vi "ex_InitTabControl.vi"(3 "DAQmx properties tree for storage":refnum<vi>, 4 "Source":refnum<vi>, 7 "error in (no error)":errorcluster, 9 "Classes":T1[](array[typedef]) {"Events"."Event Code" max=1073741823 step=1 format="%x"; "Methods"."Method Code" format="%x"; "Attributes"."Number of Dimensions" format="%x"; "Attributes"."Property Code" format="%x"}) -> ()   [LabVIEW 2020, in "Configure User Def Prop.xctl"]
uses:
  <vilib>/Platform/express/ex_EditUserDefinedProperties/Configure User Def Prop.xctl
  <vilib>/Platform/express/ex_EditUserDefinedProperties/controls.llb/ex_class3.ctl
  <vilib>/Platform/express/ex_EditUserDefinedProperties/controls.llb/ex_generictype3.ctl
  <vilib>/Platform/express/ex_EditUserDefinedProperties/controls.llb/ex_refnumenum.ctl
  <vilib>/Platform/express/ex_EditUserDefinedProperties/controls.llb/ex_cleanupenum.ctl
  <vilib>/Platform/express/ex_EditUserDefinedProperties/controls.llb/ex_yesnodefaultenum.ctl
  <vilib>/Platform/express/ex_EditUserDefinedProperties/controls.llb/ex_errorpassingenum.ctl
  <vilib>/Platform/express/ex_EditUserDefinedProperties/controls.llb/ex_matchexactenum.ctl
  <vilib>/Platform/express/ex_EditUserDefinedProperties/controls.llb/ex_callingenum.ctl
  <vilib>/Platform/express/ex_EditUserDefinedProperties/controls.llb/ex_filtering.ctl
  <vilib>/Platform/express/ex_EditUserDefinedProperties/controls.llb/ex_dialogenum.ctl
  <vilib>/Platform/express/ex_EditUserDefinedProperties/controls.llb/ex_attribute3.ctl
  <vilib>/Platform/express/ex_EditUserDefinedProperties/controls.llb/ex_datatypeenum.ctl
  <vilib>/Platform/express/ex_EditUserDefinedProperties/controls.llb/ex_clustercontrol.ctl
  <vilib>/Platform/express/ex_EditUserDefinedProperties/controls.llb/ex_enumeration.ctl
  <vilib>/Platform/express/ex_EditUserDefinedProperties/controls.llb/ex_yesnoenum.ctl
  <vilib>/Platform/express/ex_EditUserDefinedProperties/controls.llb/ex_accessenum.ctl
  <vilib>/Platform/express/ex_EditUserDefinedProperties/controls.llb/ex_initnameformat.ctl
  <vilib>/Platform/express/ex_EditUserDefinedProperties/controls.llb/ex_method3.ctl
  <vilib>/Platform/express/ex_EditUserDefinedProperties/controls.llb/ex_methflagsenum.ctl
  <vilib>/Platform/express/ex_EditUserDefinedProperties/controls.llb/ex_parameter2.ctl
  <vilib>/Platform/express/ex_EditUserDefinedProperties/controls.llb/ex_datanameenum.ctl
  <vilib>/Platform/express/ex_EditUserDefinedProperties/controls.llb/ex_numericdatatypeenum.ctl
  <vilib>/Platform/express/ex_EditUserDefinedProperties/controls.llb/ex_stringdatatypeenum.ctl
  <vilib>/Platform/express/ex_EditUserDefinedProperties/controls.llb/ex_passbyenum.ctl
  <vilib>/Platform/express/ex_EditUserDefinedProperties/controls.llb/ex_arrayfmtenum.ctl
  <vilib>/Platform/express/ex_EditUserDefinedProperties/controls.llb/ex_paraminoutenum.ctl
  <vilib>/Platform/express/ex_EditUserDefinedProperties/controls.llb/ex_eventdef.ctl
  <vilib>/Platform/express/ex_EditUserDefinedProperties/controls.llb/ex_eventparam.ctl
  <vilib>/Platform/express/ex_EditUserDefinedProperties/controls.llb/ex_eventparamtype.ctl
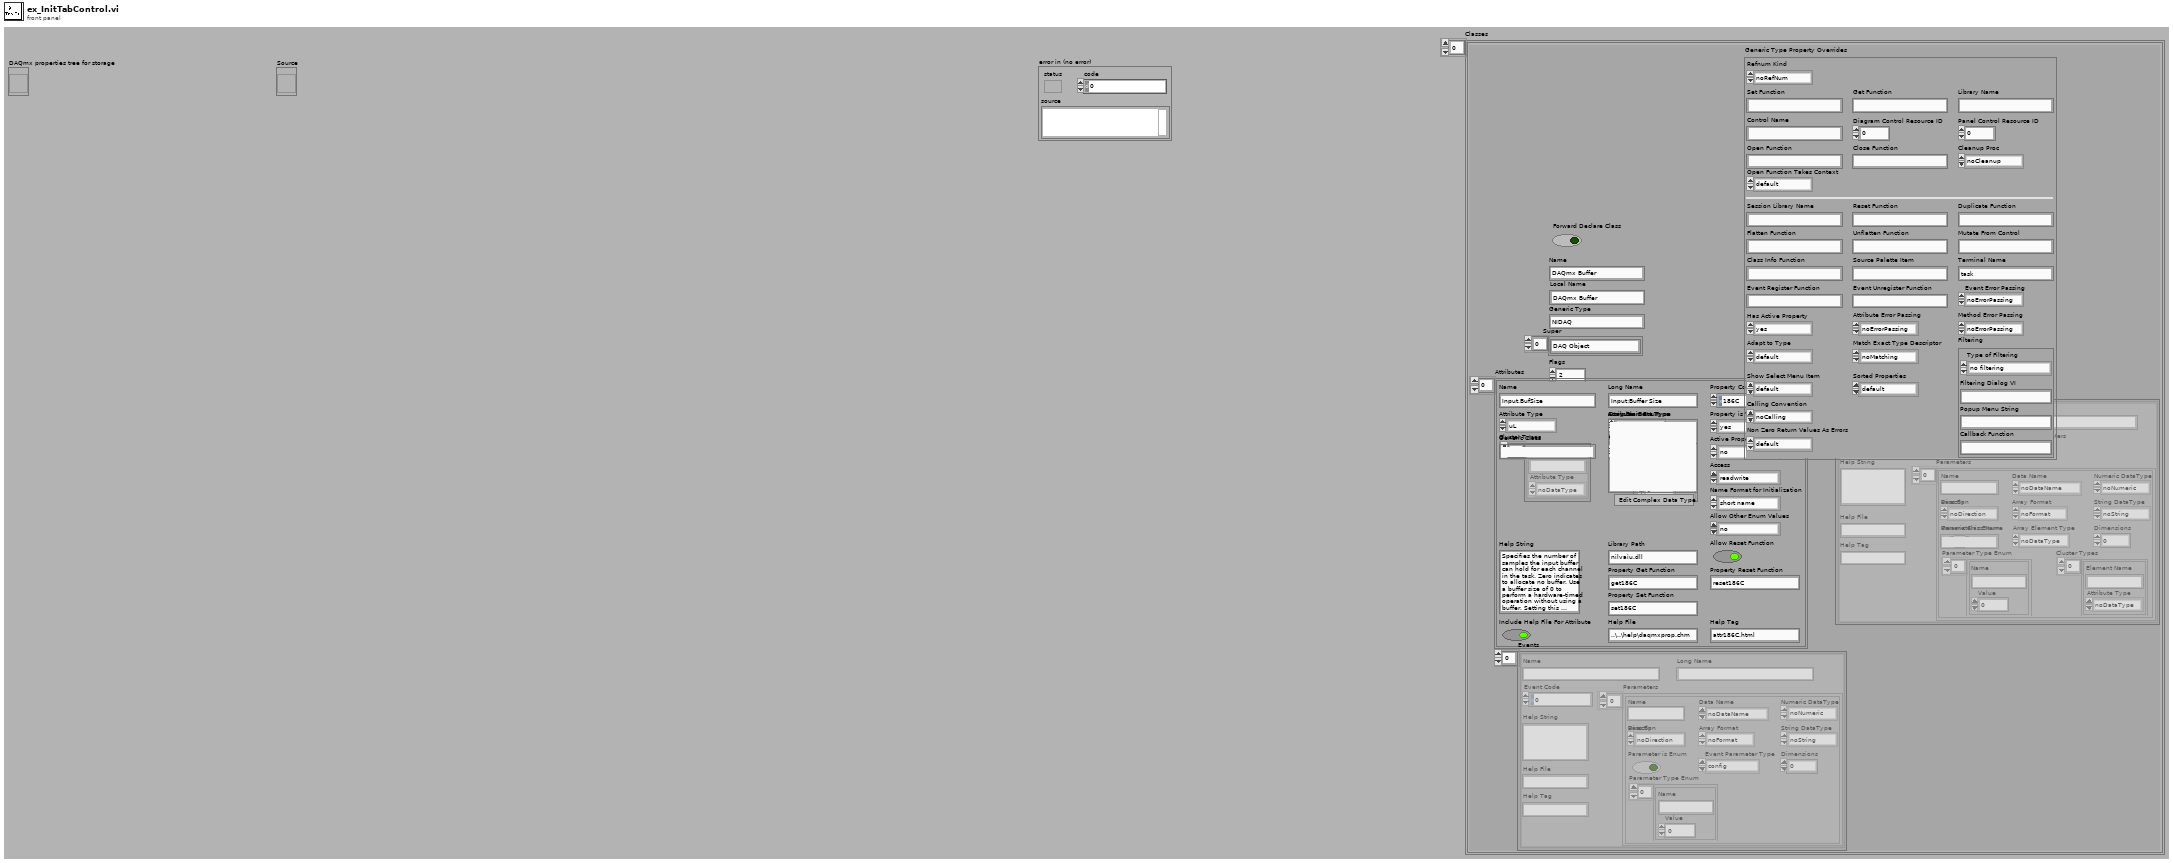
[diagram p1: front panel]
types:
  T1 = typedef "ex_class3.ctl" = cluster{"Name":string, "Local Name":string, "Generic Type":string, "Super":string[], "Forward Declare Class":bool, "Flags":i32, "Generic Type Property Overrides":T2, "Attributes":T11[], "Methods":T18[], "Events":T27[]}
  T2 = typedef "ex_generictype3.ctl" = cluster{"Refnum Kind":T3, "Set Function":string, "Get Function":string, "Library Name":string, "Control Name":string, "Diagram Control Resource ID":i32, "Panel Control Resource ID":i32, "Open Function":string, "Close Function":string, "Cleanup Proc":T4, "Open Function Takes Context":T5, "Session Library Name":string, "Reset Function":string, "Duplicate Function":string, "Flatten Function":string, "Unflatten Function":string, "Mutate From Control":string, "Class Info Function":string, "Source Palette Item":string, "Terminal Name":string, "Event Register Function":string, "Event Unregister Function":string, "Event Error Passing":T6, "Has Active Property":T5, "Attribute Error Passing":T6, "Method Error Passing":T6, "Adapt to Type":T5, "Match Exact Type Descriptor":T7, "Show Select Menu Item":T5, "Sorted Properties":T5, "Calling Convention":T8, "Filtering":T9, "Non Zero Return Values As Errors":T5}
  T3 = typedef "ex_refnumenum.ctl" = enum16{"noRefNum", "Generic", "GenericTag", "GenericByValue", "GenericByRefFlatten", "GenericTagByRefFlatten"}
  T4 = typedef "ex_cleanupenum.ctl" = enum16{"noCleanup", "exit", "idle", "reset", "idleNotTop", "resetNotTop", "doNotCleanup"}
  T5 = typedef "ex_yesnodefaultenum.ctl" = enum16{"default", "no", "yes"}
  T6 = typedef "ex_errorpassingenum.ctl" = enum16{"noErrorPassing", "none", "stringFirst", "stringLast"}
  T7 = typedef "ex_matchexactenum.ctl" = enum16{"noMatching", "none", "withInheritance", "strict"}
  T8 = typedef "ex_callingenum.ctl" = enum16{"noCalling", "std", "C"}
  T9 = typedef "ex_filtering.ctl" = cluster{"Type of Filtering":T10, "Filtering Dialog VI":string, "Popup Menu String":string, "Callback Function":string}
  T10 = typedef "ex_dialogenum.ctl" = enum16{"no filtering", "filtering", "ipfiltering"}
  T11 = typedef "ex_attribute3.ctl" = cluster{"Name":string, "Long Name":string, "Property Code":i32, "Attribute Type":T12, "Cluster Types":T13[], "Attribute is Enum":bool, "Attribute Type Enum":T14[], "Property is Visible":T15, "Active Property":T15, "Access":T16, "Help String":string, "Library Path":string, "Property Get Function":string, "Property Set Function":string, "Allow Reset Function":bool, "Property Reset Function":string, "Generic Class":string, "Allow Other Enum Values":T15, "Array Element Type":T12, "Number of Dimensions":i32, "Complex Data Type":string, "Edit Complex Data Type":bool, "Name Format for Initialization":T17, "Include Help File For Attribute":bool, "Help Tag":string, "Help File":string}
  T12 = typedef "ex_datatypeenum.ctl" = enum16{"noDataType", "void", "iB", "iW", "iL", "iQ", "uB", "uW", "uL", "uQ", "fS", "fS1D", "fD", "fD1D", "bool", "bool1D", "string", "string1D", "path", "rect", "point", "VIRef", "VIRefReservation", "file", "VIExecState", "htmlImgFmt", "printFmt", "iW1D", "uW1D", "iL1D", "uL1D", "iQ1D", "uQ1D", "uB1D", "iB1D", "VisaRef", "DAQChannel", "DAQDevice", "DAQPhysChan", "DAQScale", "DAQSwitch", "DAQTask", "DAQTerminal", "DAQTrigger", "cluster", "genclass", "timestamp", "array", "variant", "complex type"}
  T13 = typedef "ex_clustercontrol.ctl" = cluster{"Element Name":string, "Attribute Type":T12}
  T14 = typedef "ex_enumeration.ctl" = cluster{"Name":string, "Value":i32}
  T15 = typedef "ex_yesnoenum.ctl" = enum16{"no", "yes"}
  T16 = typedef "ex_accessenum.ctl" = enum16{"noAccess", "readwrite", "readonly", "writeonly"}
  T17 = typedef "ex_initnameformat.ctl" = enum16{"long name", "short name"}
  T18 = typedef "ex_method3.ctl" = cluster{"Name":string, "Local Name":string, "Method Flags":T19, "Method Code":i32, "# Optional Parameters":i32, "Parameters":T20[], "Help String":string, "Help Tag":string, "Help File":string}
  T19 = typedef "ex_methflagsenum.ctl" = enum16{"noFlags", "noInvoke", "returnValue", "returnErrClustCode", "0", "retErrClustNoInv"}
  T20 = typedef "ex_parameter2.ctl" = cluster{"Name":string, "Data Name":T21, "Numeric DataType":T22, "String DataType":T23, "Dimensions":u32, "Pass By":T24, "Array Format":T25, "Parameter is Enum":bool, "Parameter Type Enum":T14[], "Cluster Types":T13[], "Generic Class Name":string, "Array Element Type":T12, "Direction":T26}
  T21 = typedef "ex_datanameenum.ctl" = enum16{"noDataName", "numeric", "array", "string", "void", "error", "cluster", "genclass", "timestamp", "variant", "non numeric array", "bool", "path"}
  T22 = typedef "ex_numericdatatypeenum.ctl" = enum16{"noNumeric", "int8", "int16", "int32", "int64", "uInt8", "uInt16", "uInt32", "uInt64", "single", "double"}
  T23 = typedef "ex_stringdatatypeenum.ctl" = enum16{"noString", "CStr", "PStr", "StrHandle", "StrHandlePtr"}
  T24 = typedef "ex_passbyenum.ctl" = enum16{"noPassing", "value", "reference", "refInOut"}
  T25 = typedef "ex_arrayfmtenum.ctl" = enum16{"noFormat", "pointer", "handle", "handlepointer"}
  T26 = typedef "ex_paraminoutenum.ctl" = enum16{"noDirection", "in", "out", "inout"}
  T27 = typedef "ex_eventdef.ctl" = cluster{"Name":string, "Long Name":string, "Event Code":u32, "Parameters":T28[], "Help String":string, "Help Tag":string, "Help File":string}
  T28 = typedef "ex_eventparam.ctl" = cluster{"Name":string, "Data Name":T21, "Numeric DataType":T22, "String DataType":T23, "Dimensions":u32, "Pass By":T24, "Array Format":T25, "Parameter is Enum":bool, "Parameter Type Enum":T14[], "Direction":T26, "Event Parameter Type":T29}
  T29 = typedef "ex_eventparamtype.ctl" = enum16{"config", "data", "configdata"}
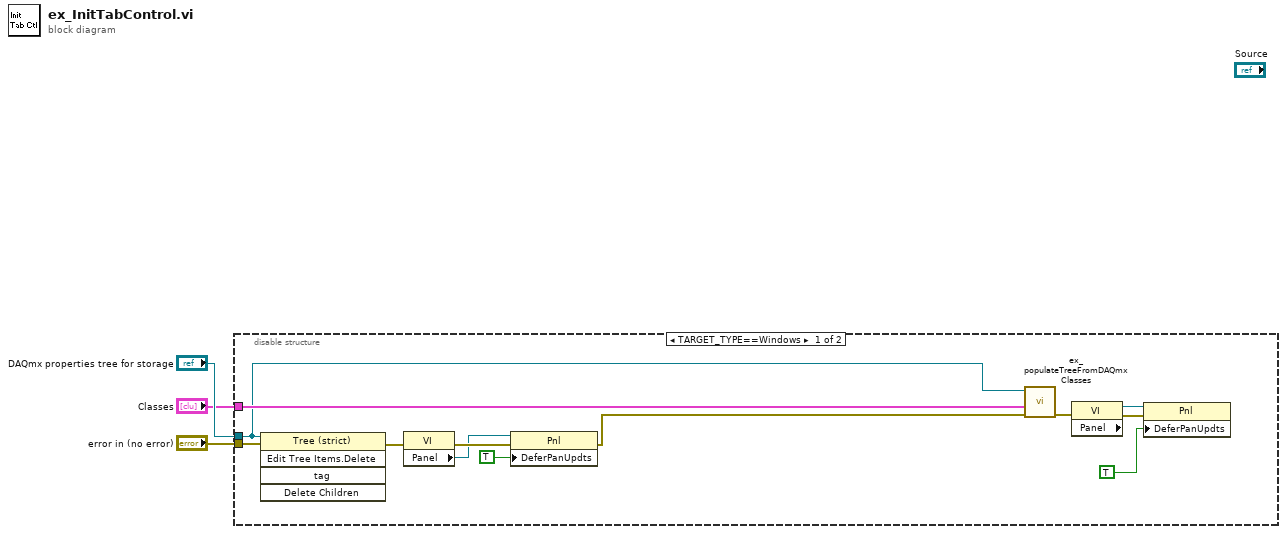
[diagram p0: block diagram]
diagram:
  n1 = disable-structure shown="TARGET_TYPE==Windows" {
    disable-tunnel: "DAQmx properties tree for storage" -> [w4 _]
    disable-tunnel: "error in (no error)" -> [w15 _]
    disable-tunnel: "Classes" -> [w5 _]
    frame condition #0 (active) {
      n2 = invoke class="Tree (strict)" method="Edit Tree Items.Delete"(reference=w4, error in=w15) -> (error out=w14:errorcluster)  [unwired: 3 in, 4 out]
      n3 = property class="VI"(error in=w14) -> (error out=w9:errorcluster, "Panel"=w8:refnum<vi>)  [unwired: 1 in, 1 out]
      n4 = property class="Pnl"(reference=w8, error in=w9, "DeferPanUpdts"=TRUE ("Defer Panel Updates")) -> (error out=w6:errorcluster)  [unwired: 1 out]
      n5 = call <vilib>:"ex_populateTreeFromDAQmxClasses.vi"("error in (no error)"=w6, "DAQmx classes"=w5, "tree ref"=w4) -> ("error out"=w13:errorcluster)  [unwired: 1 in, 3 out]
      n6 = property class="VI"(error in=w13) -> (error out=w12:errorcluster, "Panel"=w11:refnum<vi>)  [unwired: 1 in, 1 out]
      n7 = property class="Pnl"(reference=w11, error in=w12, "DeferPanUpdts"=TRUE ("Defer Panel Updates")) -> ()  [unwired: 2 out]
    }
    frame condition #1 {
    }
  }
